vi "rEAL rt tEST.vi"() -> ()   [LabVIEW 2016]
uses:
  Remote Terminal/TypeDefs/RT Configuration.ctl
  Remote Terminal/TypeDefs/Command Configuration.ctl
  Remote Terminal/TypeDefs/Command Type.ctl
  1553 SubComponent/TypeDefs/Parameter Table Data.ctl
  1553 SubComponent/TypeDefs/Scaling Information.ctl
  Remote Terminal/Remote Terminal.lvclass
  C:/SLSC 1553/Driver (Windows)/1553 SubComponent/1553 SubComponent.lvclass
  1553 Board/1553 Board.lvclass
  1553 Component/1553 Component.lvclass
  Utilities/FPGA Interface/FPGA Interface.lvclass
  1553 SubComponent/1553 SubComponent.lvclass
panel:
  out "unsigned 16bit integer":u16[][](array[numeric])
  in  "Parameter Name":string[](array[string])
  in  "Scaled Data 2":dbl[](array[numeric])
  in  "Search":bool
  in  "Read":bool
  in  "Target IC (1-8)":u8=1
  in  "Write":bool
  out "Val?":u16[](array[numeric]) format="%04x"
  in  "Val":u16[](array[numeric]) format="%04x"
  in  "Addr":u16 format="%04x"
  out "Raw Data":u64[][](array[numeric])
  out "Scaled Data":dbl[][](array[numeric])
  out "Parameters":string[][](array[string])
  in  "stop":bool
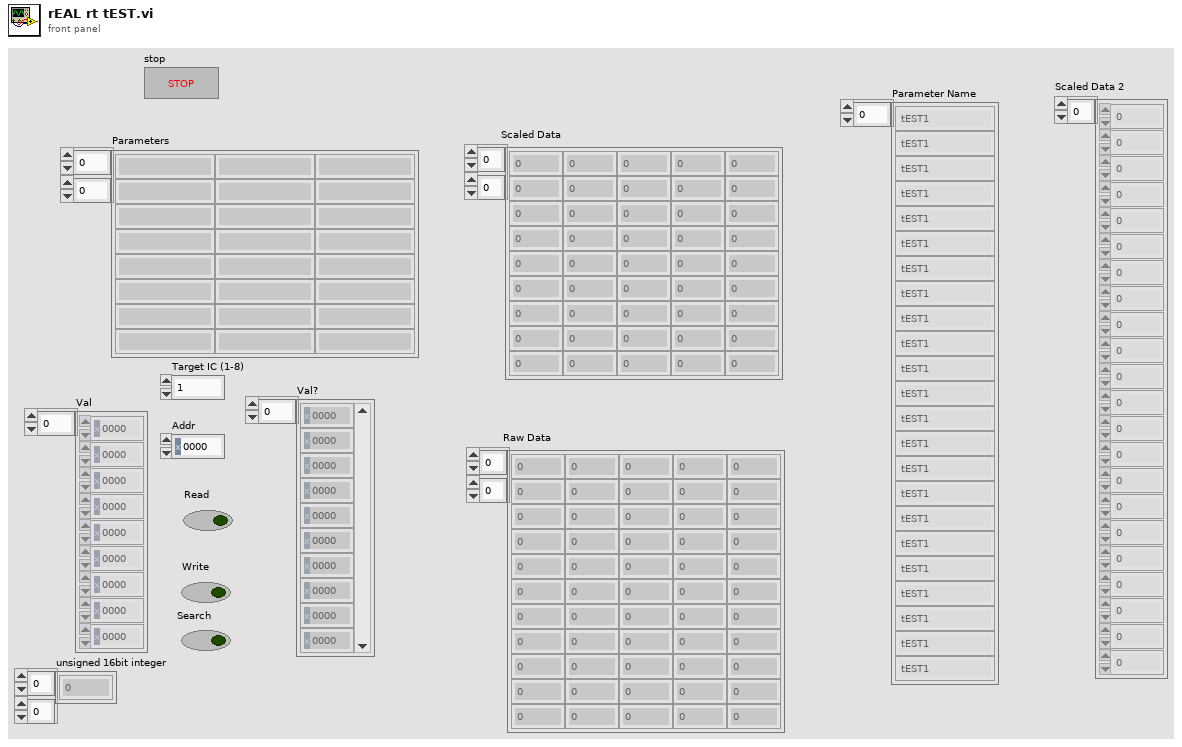
[diagram p1: front panel]
types:
  T1 = typedef "SLSC 1553 API.lvlib/1553 SubComponent.lvclass/Parameter Table Data.ctl" = cluster{"Parameter Name":string, "Base Word":u16, "Address":u16, "Value":u64, "Mask":u16[], "Scaling Info":T2}
  T2 = typedef "SLSC 1553 API.lvlib/1553 SubComponent.lvclass/Scaling Information.ctl" = cluster{"Bit Offset":i32, "Bit Count":i32, "LSB Resolution":dbl, "2's Complement":bool, "Big Endian":bool}
  T3 = typedef "SLSC 1553 API.lvlib/Remote Terminal.lvclass/Command Type.ctl" = enum16{"Transmit", "Receive", "Mode Code Tx", "Mode Code Rx"}
  T4 = typedef "SLSC 1553 API.lvlib/Remote Terminal.lvclass/Command Configuration.ctl" = cluster{"Command Type":T3, "Mode Code ID (1-32)":u16, "SubAddress (1-30)":u16, "Word Count (1-32)":u16, "Illegal Command":bool, "Broadcast":bool, "Data":u16[], "Data Fields":T1[]}
  T5 = typedef "SLSC 1553 API.lvlib/Remote Terminal.lvclass/RT Configuration.ctl" = cluster{"RT-RT TimeOut (us)":u8, "Inhibit Bus A":bool, "Inhibit Bus B":bool, "Broadcast CMD Invalid":bool, "UnDef MCs Invalid":bool, "Notice 2 Data Storage":bool, "SMCP":bool, "Temp RX Buffer":bool, "Alt BIT Enable":bool, "Auto Bus Shutdown":bool, "MC 17 Sync":u8, "MC 16 SR Reset":bool, "MC 8 Reset":bool}
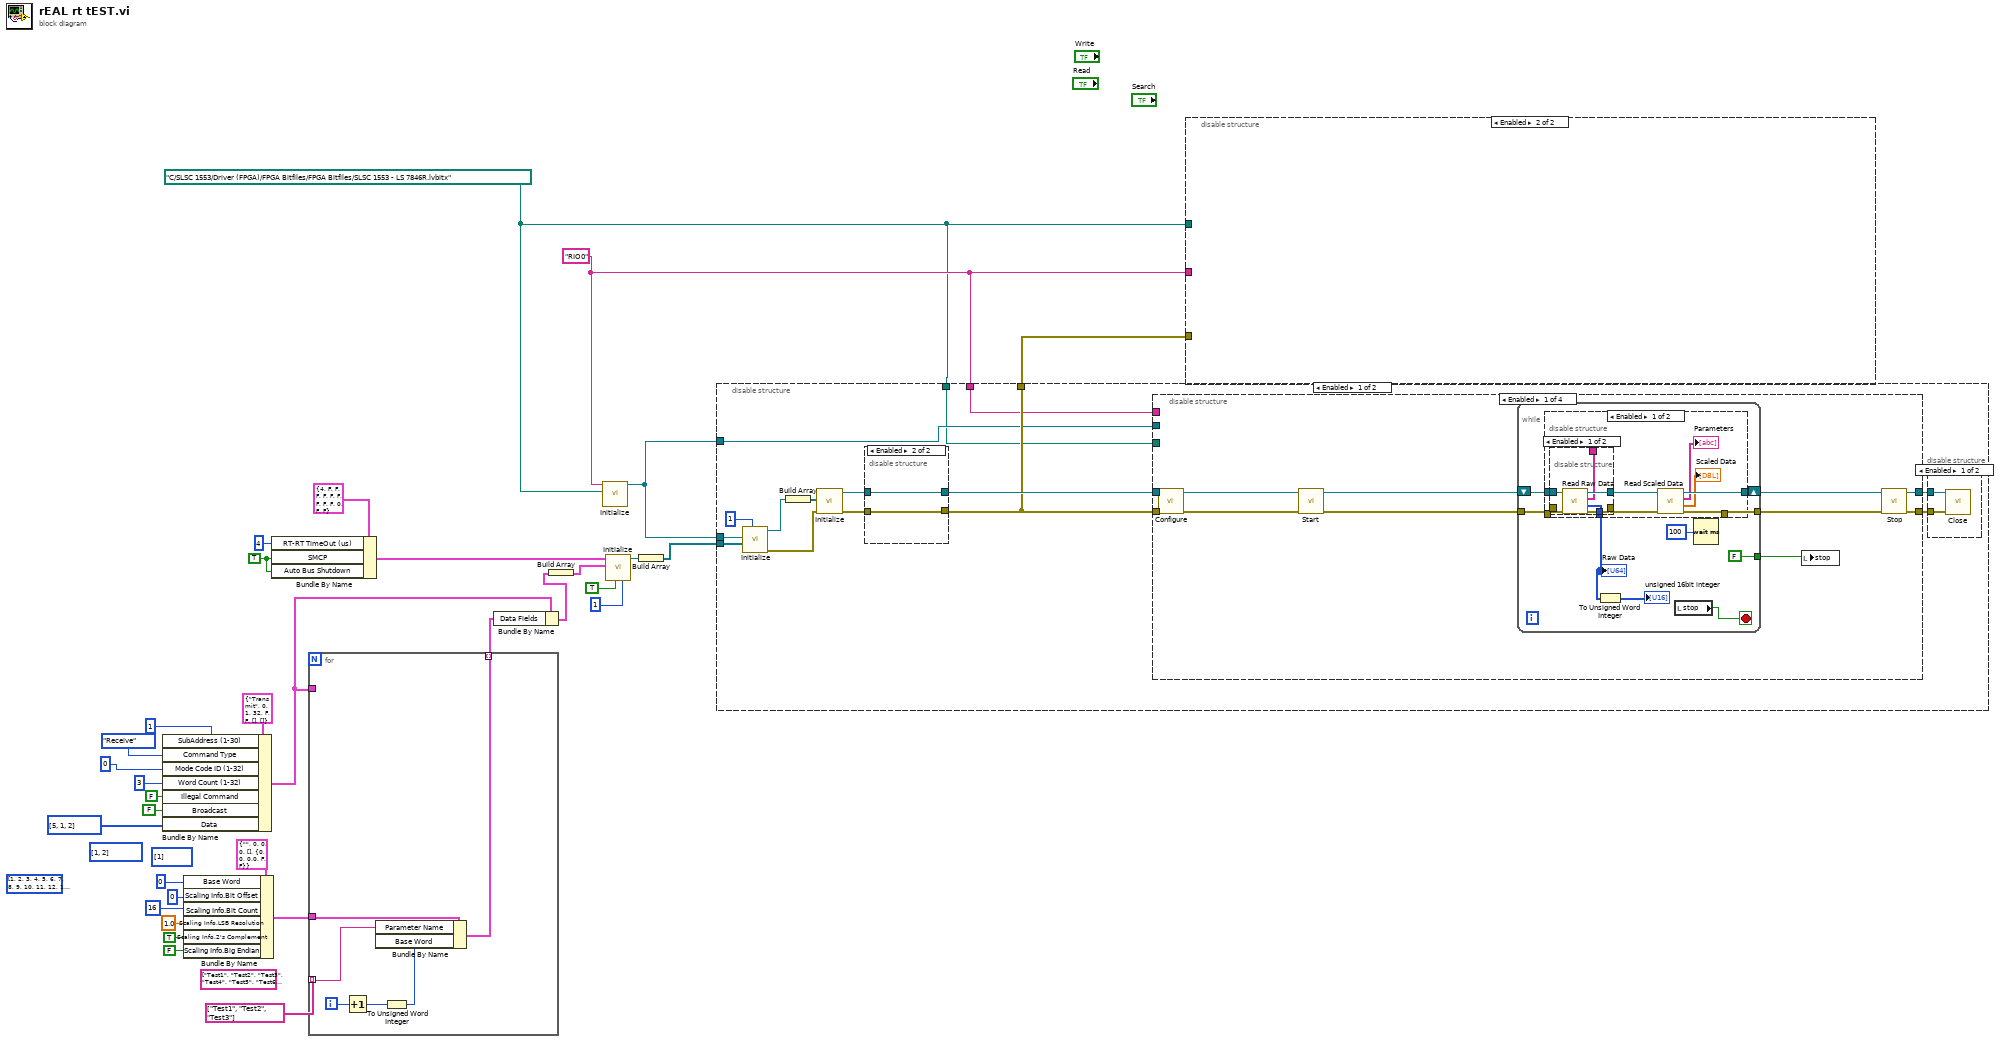
[diagram p0: block diagram]
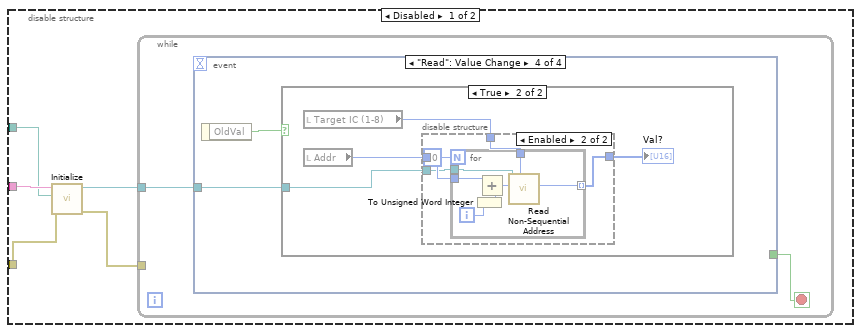
[diagram p2: hidden frame]
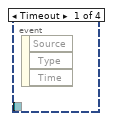
[diagram p3: hidden frame]
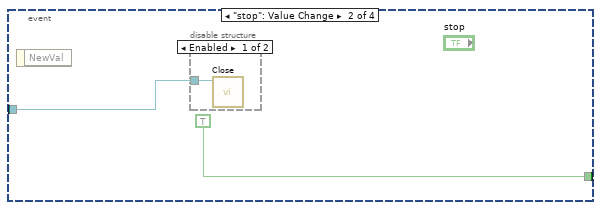
[diagram p4: hidden frame]
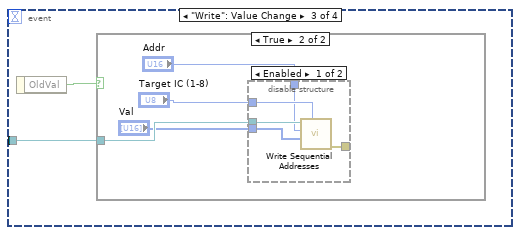
[diagram p6: hidden frame]
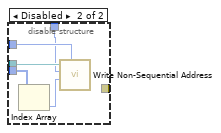
[diagram p8: hidden frame]
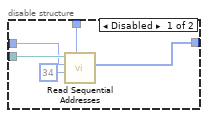
[diagram p10: hidden frame]
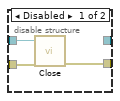
[diagram p12: hidden frame]
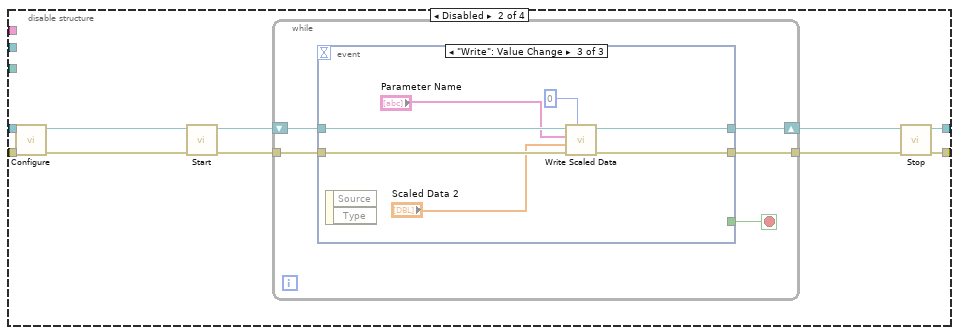
[diagram p15: hidden frame]
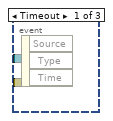
[diagram p16: hidden frame]
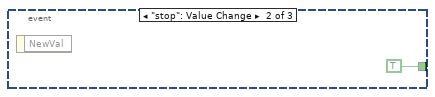
[diagram p17: hidden frame]
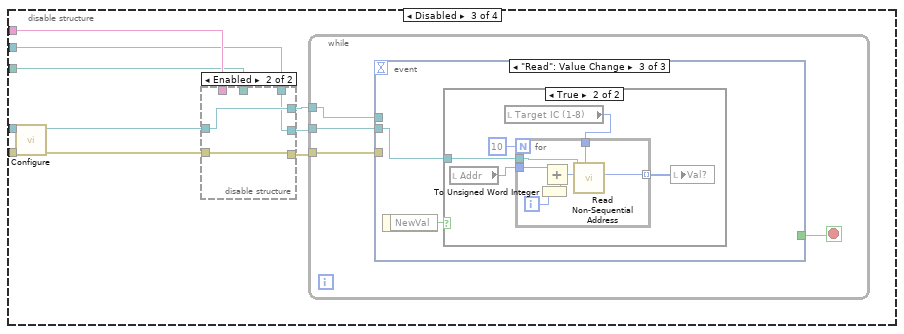
[diagram p18: hidden frame]
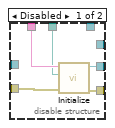
[diagram p19: hidden frame]
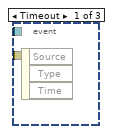
[diagram p20: hidden frame]
diagram:
  (unwired) u16[] [1] ("Data")
  (unwired) u16[] [1, 2] ("Data")
  (unwired) string[] ["Test1", "Test2", "Test3", "Test4", "Test5", "Test6", "Test7", "Test8", "Test9", "Test10", "Test11", "Test12", "Test13", "Test14", "Test15", "Test16", "Test17", "Test18", "Test19", "Test20", "Test21", "Test22", "Test23", "Test24", "Test25", "Test26", "Test27", "Test28", "Test29", "Test30"] ("Parameter Name")
  (unwired) u16[] [1, 2, 3, 4, 5, 6, 7, 8, 9, 10, 11, 12, 13, 14, 15, 16, 17, 18, 19, 20, 21, 22, 23, 24, 25, 32] ("Data")
  w11 = path "C:/SLSC 1553/Driver (FPGA)/FPGA Bitfiles/FPGA Bitfiles/SLSC 1553 - LS 7846R.lvbitx" ("Bitfile path")
  w12 = "RIO0" ("Device address")
  w32 = TRUE ("SMCP")
  n1 = Bundle By Name(cluster=T4 {"Command Type"=enum."Transmit", "Mode Code ID (1-32)"=0, "SubAddress (1-30)"=1, "Word Count (1-32)"=32, "Illegal Command"=FALSE, "Broadcast"=FALSE, "Data"=[], "Data Fields"=[]} ("CMD Configuration"), "SubAddress (1-30)"=u16 1, "Command Type"=Command_Type."Receive", "Mode Code ID (1-32)"=u16 0, "Word Count (1-32)"=u16 3, "Illegal Command"=FALSE, "Broadcast"=FALSE, "Data"=u16[] [5, 1, 2]) -> (w5:T4)
  n2 = Bundle By Name(cluster=T1 {"Parameter Name"="", "Base Word"=0, "Address"=0, "Value"=0, "Mask"=[], "Scaling Info"={"Bit Offset"=0, "Bit Count"=0, "LSB Resolution"=0.0, "2's Complement"=FALSE, "Big Endian"=FALSE}} ("Parameter Table Data"), "Base Word"=u16 0, "Scaling Info.Bit Offset"=0, "Scaling Info.Bit Count"=16, "Scaling Info.LSB Resolution"=1.0, "Scaling Info.2's Complement"=TRUE, "Scaling Info.Big Endian"=FALSE) -> (w8:T1)
  n3 = Bundle By Name(cluster=T5 {"RT-RT TimeOut (us)"=4, "Inhibit Bus A"=FALSE, "Inhibit Bus B"=FALSE, "Broadcast CMD Invalid"=FALSE, "UnDef MCs Invalid"=FALSE, "Notice 2 Data Storage"=FALSE, "SMCP"=FALSE, "Temp RX Buffer"=FALSE, "Alt BIT Enable"=FALSE, "Auto Bus Shutdown"=FALSE, "MC 17 Sync"=0, "MC 16 SR Reset"=FALSE, "MC 8 Reset"=FALSE} ("RT Configuration"), "RT-RT TimeOut (us)"=u8 4, "SMCP"=w32, "Auto Bus Shutdown"=w32) -> (w27:T5)
  n4 = for {
    tunnel: w5 -> [_]
    tunnel: string[] ["Test1", "Test2", "Test3"] ("Parameter Name") -> [w36] mode=indexing
    tunnel: w8 -> [w37]
    tunnel: [w34] -> w4 mode=indexing
    i -> [w39]
    n5 = Increment(x=w39) -> (x+1=w38:i32)
    n6 = To Unsigned Word Integer(number=w38) -> (unsigned 16bit integer=w35:u16)
    n7 = Bundle By Name(cluster=w37, "Parameter Name"=w36, "Base Word"=w35) -> (w34:T1)
  }
  n8 = Bundle By Name(cluster=w5, "Data Fields"=w4) -> (w3:T4)
  n9 = Build Array(w3) -> (w2:T4[])
  n10 = call "Initialize.vi"("Bitfile path"=w11, "Device address"=w12) -> ("FPGA Interface out"=w13:refnum<class "FPGA Interface.lvclass">)  [unwired: 8 in, 1 out]
  n11 = call "Initialize.vi"("RT Address (0-30)"=u8 1, "RT 1?"=TRUE, "Commands"=w2, "RT Configuration"=w27) -> ("Remote Terminal out"=w26:refnum<class "Remote Terminal.lvclass">)  [unwired: 6 in, 1 out]
  n12 = Build Array(w26) -> (w33:refnum<class "Remote Terminal.lvclass">[])
  n13 = disable-structure shown="Enabled" {
    disable-tunnel: w33 -> [w54 _]
    disable-tunnel: w13 -> [w53 _]
    disable-tunnel: [w45 _] -> w14
    disable-tunnel: w13 -> [w42 _]
    disable-tunnel: w12 -> [w41 _]
    disable-tunnel: w11 -> [w40 _]
    frame Enabled {
      n14 = call "Initialize.vi"("Component ID (1-8)"=u8 1 ("Component ID"), "SubComponents"=w54, "FPGA Interface"=w53) -> ("error out"=w51:errorcluster, "1553 Component out"=w50:refnum<class "1553 Component.lvclass">)  [unwired: 7 in]
      n15 = Build Array(w50) -> (w49:refnum<class "1553 Component.lvclass">[])
      n16 = call "Initialize.vi"("error in (no error)"=w51, "Components"=w49) -> ("error out"=w48:errorcluster, "1553 Board out"=w47:refnum<class "1553 Board.lvclass">)  [unwired: 8 in]
      n17 = disable-structure shown="Enabled" {
        disable-tunnel: [w59 w61] -> w45
        disable-tunnel: w48 -> [w58 w61]
        disable-tunnel: w47 -> [w57 w60]
        disable-tunnel: [_ w60] -> w46
        frame Disabled {
          n18 = call-dynamic "Close.vi"("error in (no error)"=w58, "1553 Board in"=w57) -> ("error out"=w59:errorcluster)  [unwired: 9 in]
        }
        frame Enabled {
        }
      }
      n19 = disable-structure shown="Enabled" {
        disable-tunnel: w46 -> [w72 w109 w132 _]
        disable-tunnel: w45 -> [w71 w108 w131 _]
        disable-tunnel: [w65 w102 _ _] -> w44
        disable-tunnel: [w64 w101 _ _] -> w43
        disable-tunnel: w42 -> [_ _ w123 _]
        disable-tunnel: w41 -> [_ _ w128 _]
        disable-tunnel: w40 -> [_ _ w127 _]
        frame Enabled {
          n20 = call-dynamic "Configure.vi"("error in (no error)"=w71, "1553 Board in"=w72) -> ("error out"=w69:errorcluster, "1553 Board out"=w70:refnum<class "1553 Board.lvclass">)  [unwired: 8 in]
          n21 = call-dynamic "Start.vi"("error in (no error)"=w69, "1553 Board in"=w70) -> ("error out"=w66:errorcluster, "1553 Board out"=w68:refnum<class "1553 Board.lvclass">)  [unwired: 8 in]
          n22 = while {
            shift-right: [w79] -> w63
            shift-left: w68 -> [w77]
            tunnel: [w80] -> w67
            tunnel: w66 -> [w78]
            tunnel: [FALSE] -> w62
            stop <- w76 stop-if-true
            n23 = disable-structure shown="Enabled" {
              disable-tunnel: [w90 _] -> w80
              disable-tunnel: [w89 w99] -> w79
              disable-tunnel: w78 -> [w87 _]
              disable-tunnel: w77 -> [w86 w99]
              disable-tunnel: [w83 _] -> w74
              frame Enabled {
                n24 = disable-structure shown="Enabled" {
                  disable-tunnel: w87 -> [w96 w97]
                  disable-tunnel: w86 -> [w95 w98]
                  disable-tunnel: [w94 w98] -> w85
                  disable-tunnel: [w93 w97] -> w84
                  disable-tunnel: [w92 _] -> _
                  disable-tunnel: [w91 _] -> w83
                  frame Enabled {
                    n25 = call-dynamic "Read Raw Data.vi"("error in (no error)"=w96, "1553 Board in"=w95) -> ("error out"=w93:errorcluster, "Raw Data"=w91:u64[][], "Parameters"=w92:string[][], "1553 Board out"=w94:refnum<class "1553 Board.lvclass">)  [unwired: 6 in]
                  }
                  frame Disabled {
                  }
                }
                n26 = call-dynamic "Read Scaled Data.vi"("error in (no error)"=w84, "1553 Board in"=w85) -> ("error out"=w90:errorcluster, "Scaled Data"=→"Scaled Data":dbl[][], "Parameters"=→"Parameters":string[][], "1553 Board out"=w89:refnum<class "1553 Board.lvclass">)  [unwired: 6 in]
              }
              frame Disabled {
              }
            }
            "Raw Data" <- w74
            n27 = To Unsigned Word Integer(number=w74) -> (unsigned 16bit integer=→"unsigned 16bit integer":u16[][])
            n28 = local read "stop"() -> (w76:bool)
            n29 = Wait (ms)(milliseconds to wait=u32 100) -> ()  [unwired: 1 out]
          }
          n30 = local write "stop"(w62) -> ()
          n31 = call-dynamic "Stop.vi"("error in (no error)"=w67, "1553 Board in"=w63) -> ("error out"=w65:errorcluster, "1553 Board out"=w64:refnum<class "1553 Board.lvclass">)  [unwired: 8 in]
        }
        frame Disabled {
          n32 = call-dynamic "Configure.vi"("error in (no error)"=w108, "1553 Board in"=w109) -> ("error out"=w106:errorcluster, "1553 Board out"=w107:refnum<class "1553 Board.lvclass">)  [unwired: 8 in]
          n33 = call-dynamic "Start.vi"("error in (no error)"=w106, "1553 Board in"=w107) -> ("error out"=w103:errorcluster, "1553 Board out"=w105:refnum<class "1553 Board.lvclass">)  [unwired: 8 in]
          n34 = while {
            shift-right: [w110] -> w100
            shift-left: w105 -> [w112]
            tunnel: [w111] -> w104
            tunnel: w103 -> [w113]
            stop <- w114 stop-if-true
            n35 = event shown="[2] \"Write\": Value Change" {
              selector: _ -> [_ _ _]
              dyn-events: _ -> [_ _ _]
              timeout: _ -> [_ _ _]
              tunnel: [_ TRUE _] -> w114
              tunnel: w113 -> [_ _ w122]
              tunnel: w112 -> [_ _ w121]
              tunnel: [_ _ w119] -> w111
              tunnel: [_ _ w118] -> w110
              event Timeout {
                n36 = event-data() -> ()  [unwired: 1 in, 3 out]
              }
              event "stop": Value Change {
                n37 = event-data() -> ()  [unwired: 1 in, 1 out]
              }
              event "Write": Value Change {
                n38 = event-data() -> ()  [unwired: 1 in, 2 out]
                n39 = call-dynamic "Write Scaled Data.vi"("Component Index"=0, "error in (no error)"=w122, "Scaled Data"="Scaled Data 2", "Parameters"="Parameter Name", "1553 Board in"=w121) -> ("error out"=w119:errorcluster, "1553 Board out"=w118:refnum<class "1553 Board.lvclass">)  [unwired: 5 in]
              }
            }
          }
          n40 = call-dynamic "Stop.vi"("error in (no error)"=w104, "1553 Board in"=w100) -> ("error out"=w102:errorcluster, "1553 Board out"=w101:refnum<class "1553 Board.lvclass">)  [unwired: 8 in]
        }
        frame Disabled {
          n41 = call-dynamic "Configure.vi"("error in (no error)"=w131, "1553 Board in"=w132) -> ("error out"=w126:errorcluster, "1553 Board out"=w125:refnum<class "1553 Board.lvclass">)  [unwired: 8 in]
          n42 = disable-structure shown="Enabled" {
            disable-tunnel: [w137 w140] -> w130
            disable-tunnel: [w136 w138] -> w129
            disable-tunnel: w128 -> [w135 _]
            disable-tunnel: w127 -> [w134 _]
            disable-tunnel: w126 -> [w133 w140]
            disable-tunnel: w125 -> [_ w139]
            disable-tunnel: [_ w139] -> w124
            disable-tunnel: w123 -> [_ w138]
            frame Disabled {
              n43 = call "Initialize.vi"("error in (no error)"=w133, "Bitfile path"=w134, "Device address"=w135) -> ("error out"=w137:errorcluster, "FPGA Interface out"=w136:refnum<class "FPGA Interface.lvclass">)  [unwired: 7 in]
            }
            frame Enabled {
            }
          }
          n44 = while {
            tunnel: w130 -> [w143]
            tunnel: w129 -> [w142]
            tunnel: w124 -> [w141]
            stop <- w144 stop-if-true
            n45 = event shown="[2] \"Read\": Value Change" {
              selector: _ -> [_ _ _]
              dyn-events: _ -> [_ _ _]
              timeout: _ -> [_ _ _]
              tunnel: [_ TRUE _] -> w144
              tunnel: w143 -> [_ w147 _]
              tunnel: w142 -> [_ w146 w153]
              tunnel: w141 -> [_ w145 _]
              event Timeout {
                n46 = event-data() -> ()  [unwired: 1 in, 3 out]
              }
              event "stop": Value Change {
                n47 = event-data() -> ()  [unwired: 1 in, 1 out]
                n48 = disable-structure shown="Enabled" {
                  disable-tunnel: w147 -> [w150 w152]
                  disable-tunnel: w146 -> [w149 _]
                  disable-tunnel: w145 -> [_ w151]
                  frame Disabled {
                    n49 = call "Close.vi"("error in (no error)"=w150, "FPGA Interface in"=w149) -> ()  [unwired: 9 in, 1 out]
                  }
                  frame Enabled {
                    n50 = call-dynamic "Close.vi"("error in (no error)"=w152, "1553 Board in"=w151) -> ()  [unwired: 9 in, 1 out]
                  }
                }
              }
              event "Read": Value Change {
                n51 = event-data() -> ("NewVal"=w154:bool)  [unwired: 1 in]
                n52 = case shown="True" w154 {
                  tunnel: w153 -> [_ w159]
                  frame False {
                  }
                  frame True {
                    n53 = local read "Addr"() -> (w157:u16)
                    n54 = local read "Target IC (1-8)"() -> (w158:u8)
                    n55 = for {
                      N: 10 -> [_]
                      tunnel: w157 -> [w162]
                      tunnel: w159 -> [w166]
                      tunnel: w158 -> [w165]
                      tunnel: [w164] -> w156 mode=indexing
                      i -> [w161]
                      n56 = To Unsigned Word Integer(number=w161) -> (unsigned 16bit integer=w160:u16)
                      n57 = Add(x=w162, y=w160) -> (x+y=w163:u16)
                      n58 = call-dynamic "Read Non-Sequential Address.vi"("Target IC (1-8)"=w165, "Address"=w163, "FPGA Interface in"=w166) -> ("Data"=w164:u16)  [unwired: 7 in, 1 out]
                    }
                    n59 = local write "Val?"(w156) -> ()
                  }
                }
              }
            }
          }
        }
        frame Disabled {
        }
      }
      n60 = disable-structure shown="Enabled" {
        disable-tunnel: w44 -> [w56 _]
        disable-tunnel: w43 -> [w55 _]
        frame Enabled {
          n61 = call-dynamic "Close.vi"("error in (no error)"=w56, "1553 Board in"=w55) -> ()  [unwired: 9 in, 1 out]
        }
        frame Disabled {
        }
      }
    }
    frame Disabled {
    }
  }
  n62 = disable-structure shown="Enabled" {
    disable-tunnel: w14 -> [w171 _]
    disable-tunnel: w12 -> [w170 _]
    disable-tunnel: w11 -> [w169 _]
    frame Disabled {
      n63 = call "Initialize.vi"("error in (no error)"=w171, "Bitfile path"=w169, "Device address"=w170) -> ("error out"=w168:errorcluster, "FPGA Interface out"=w167:refnum<class "FPGA Interface.lvclass">)  [unwired: 7 in]
      n64 = while {
        tunnel: w167 -> [w173]
        tunnel: w168 -> [_]
        stop <- w172 stop-if-true
        n65 = event shown="[3] \"Read\": Value Change" {
          selector: _ -> [_ _ _ _]
          dyn-events: _ -> [_ _ _ _]
          timeout: _ -> [_ _ _ _]
          tunnel: w173 -> [_ w174 w177 w193]
          tunnel: [_ TRUE _ _] -> w172
          event Timeout {
            n66 = event-data() -> ()  [unwired: 1 in, 3 out]
          }
          event "stop": Value Change {
            n67 = event-data() -> ()  [unwired: 1 in, 1 out]
            n68 = disable-structure shown="Enabled" {
              disable-tunnel: w174 -> [w176 _]
              frame Enabled {
                n69 = call "Close.vi"("FPGA Interface in"=w176) -> ()  [unwired: 10 in, 1 out]
              }
              frame Disabled {
              }
            }
          }
          event "Write": Value Change {
            n70 = event-data() -> ("OldVal"=w178:bool)  [unwired: 1 in]
            n71 = case shown="True" w178 {
              tunnel: w177 -> [_ w182]
              frame False {
              }
              frame True {
                n72 = disable-structure shown="Enabled" {
                  disable-tunnel: w182 -> [w187 w192]
                  disable-tunnel: "Target IC (1-8)" -> [w186 w191]
                  disable-tunnel: [w185 _] -> _
                  disable-tunnel: "Addr" -> [w184 w190]
                  disable-tunnel: "Val" -> [w183 w189]
                  frame Enabled {
                    n73 = call-dynamic "Write Sequential Addresses.vi"("Target IC (1-8)"=w186, "Data"=w183, "Starting Address"=w184, "FPGA Interface in"=w187) -> ("error out"=w185:errorcluster)  [unwired: 7 in]
                  }
                  frame Disabled {
                    n74 = Index Array(array=w189) -> (element=w188:u16)  [unwired: 1 in]
                    n75 = call-dynamic "Write Non-Sequential Address.vi"("Target IC (1-8)"=w191, "Data"=w188, "Address"=w190, "FPGA Interface in"=w192) -> ()  [unwired: 7 in, 1 out]
                  }
                }
              }
            }
          }
          event "Read": Value Change {
            n76 = event-data() -> ("OldVal"=w194:bool)  [unwired: 1 in]
            n77 = case shown="True" w194 {
              tunnel: w193 -> [_ w197]
              frame False {
              }
              frame True {
                n78 = local read "Target IC (1-8)"() -> (w195:u8)
                n79 = local read "Addr"() -> (w196:u16)
                n80 = disable-structure shown="Enabled" {
                  disable-tunnel: [w203 w205] -> w198
                  disable-tunnel: w197 -> [w201 w207]
                  disable-tunnel: w196 -> [w200 w208]
                  disable-tunnel: w195 -> [w199 w206]
                  frame Disabled {
                    n81 = call-dynamic "Read Sequential Addresses.vi"("Target IC (1-8)"=w199, "Addresses to Read"=u16 34, "Starting Address"=w200, "FPGA Interface in"=w201) -> ("Data"=w203:u16[])  [unwired: 6 in, 1 out]
                  }
                  frame Enabled {
                    n82 = for {
                      N: 10 -> [_]
                      tunnel: w208 -> [w211]
                      tunnel: w207 -> [w215]
                      tunnel: w206 -> [w214]
                      tunnel: [w213] -> w205 mode=indexing
                      i -> [w210]
                      n83 = To Unsigned Word Integer(number=w210) -> (unsigned 16bit integer=w209:u16)
                      n84 = Add(x=w211, y=w209) -> (x+y=w212:u16)
                      n85 = call-dynamic "Read Non-Sequential Address.vi"("Target IC (1-8)"=w214, "Address"=w212, "FPGA Interface in"=w215) -> ("Data"=w213:u16)  [unwired: 7 in, 1 out]
                    }
                  }
                }
                "Val?" <- w198
              }
            }
          }
        }
      }
    }
    frame Enabled {
    }
  }
